vi "Clear Task Wrapper.vi"(0 "Task map in":map{string, refnum<k21>}(c390), 5 "Message Data in":T2, 11 "error in (no error)":errorcluster) -> (4 "Task map out":map{string, refnum<k21>}(c390), 6 "Message Data out":T1, 15 "error out":errorcluster)   [LabVIEW 2021, in "NI DAQmx_wrapper.lvlib"]
uses:
  NI DAQmx_wrapper.lvlib
  NI DAQmx_server/RPC Messages/nidaqmx_grpc_ClearTaskRequest.ctl
  NI DAQmx_server/RPC Messages/nidevice_grpc_Session_session/nidevice_grpc_Session_session.lvclass
  NI DAQmx_server/RPC Messages/nidevice_grpc_Session.ctl
  NI DAQmx_server/RPC Messages/nidaqmx_grpc_ClearTaskResponse.ctl
  NI DAQmx_server/RPC Messages/nidevice_grpc_Session_session/nidevice_grpc_Session_session.lvclass/nidevice_grpc_Session_session.ctl
  NI DAQmx_server/NI DAQmx_server.lvlib
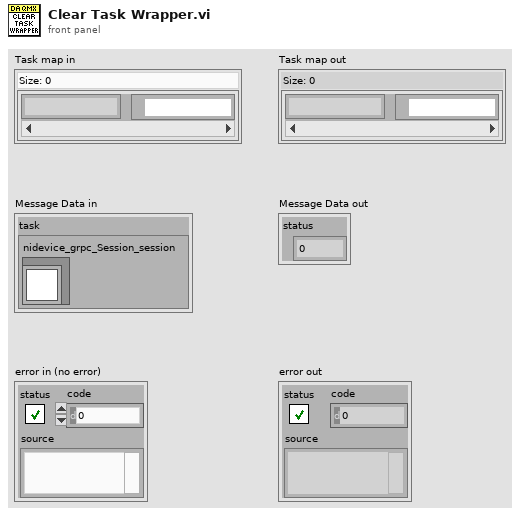
[diagram p1: front panel]
types:
  T1 = typedef "NI DAQmx_server.lvlib/nidaqmx_grpc_ClearTaskResponse.ctl" = cluster{"status":i32}
  T2 = typedef "NI DAQmx_server.lvlib/nidaqmx_grpc_ClearTaskRequest.ctl" = cluster{"task":T3}
  T3 = typedef "NI DAQmx_server.lvlib/nidevice_grpc_Session.ctl" = cluster{"nidevice_grpc_Session_session":refnum<class "nidevice_grpc_Session_session.lvclass">}
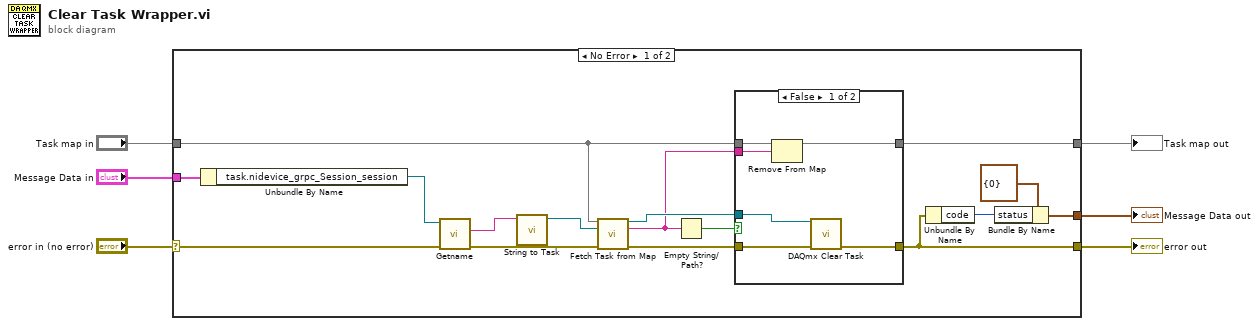
[diagram p0: block diagram]
diagram:
  n1 = case shown="No Error" "error in (no error)" {
    selector: "error in (no error)" -> [w20 w32]
    tunnel: "Task map in" -> [w12 w31]
    tunnel: "Message Data in" -> [w22 _]
    tunnel: [w10 w32] -> w3
    tunnel: [w11 w31] -> w2
    tunnel: [w7 _] -> w1
    frame No Error {
      n2 = Unbundle By Name(w22) -> ("task.nidevice_grpc_Session_session"=w21:refnum<class "nidevice_grpc_Session_session.lvclass">)
      n3 = call "Getname.vi"("error in (no error)"=w20, "OneOfTemplate in"=w21) -> ("error out"=w18:errorcluster, "Get_Val"=w17:string)  [unwired: 7 in, 1 out]
      n4 = call "String to Task.vi"("Get_Val"=w17) -> ("Refnum out"=w19:refnum<k21>)  [unwired: 10 in]
      n5 = call "Fetch Task from Map.vi"("Task map in"=w12, "Task in"=w19, "error in (no error)"=w18) -> ("Task out"=w14:refnum<k21>, "Session Name"=w13:string, "error out"=w16:errorcluster)  [unwired: 10 in]
      n6 = Empty String/Path?(string/path=w13) -> (empty?=w15:bool)
      n7 = case shown="False" w15 {
        tunnel: w16 -> [w28 w29]
        tunnel: w14 -> [w23 _]
        tunnel: [w27 w29] -> w10
        tunnel: w13 -> [w25 _]
        tunnel: w12 -> [w26 w30]
        tunnel: [w24 w30] -> w11
        frame False {
          n8 = Remove From Map(10:w25, 11:w26) -> (3:w24:map{string, refnum<k21>})  [unwired: 2 out]
          n9 = call <vilib>:"DAQmx Clear Task.vi"("task in"=w23, "error in"=w28) -> ("error out"=w27:errorcluster)  [unwired: 13 in]
        }
        frame True {
        }
      }
      n10 = Unbundle By Name(w10) -> ("code"=w8:i32)
      n11 = Bundle By Name(cluster=T1 {"status"=0} ("Message Data 2"), "status"=w8) -> (w7:T1)
    }
    frame Error {
    }
  }
  "error out" <- w3
  "Task map out" <- w2
  "Message Data out" <- w1
